vi "FPGA_target_find_stop_output.vi"(5 "start_addr":u32, 7 "number_cmds_in":u32) -> (9 "C0_data":T1, 10 "found":bool, 11 "C1_data":T1, 13 "number_cmds_dup":u32)   [LabVIEW 2014]
doc: "This VI searchs the next stop command following the start address."
uses:
  FPGA_32BitPattern_data_type.ctl
  <vilib>/rvi/Emulation/niFpgaCriticalErrorInLSC.vi
  <vilib>/rvi/Emulation/niFpgaEmulationReportErrorSimple.vi
  <vilib>/rvi/Emulation/niFpgaSctlEmulationGetInTimedLoop.vi
  <vilib>/rvi/Emulation/niFpgaGetClockAttributes.vi
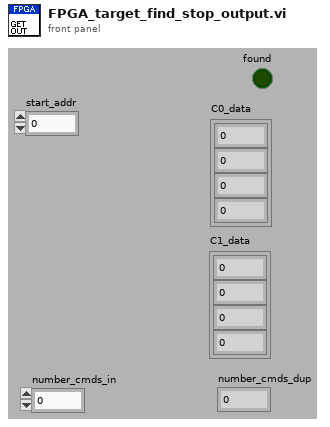
[diagram p1: front panel]
types:
  T1 = typedef "FPGA_32BitPattern_data_type.ctl" = cluster{"port0":u8, "port1":u8, "port2":u8, "port3":u8}
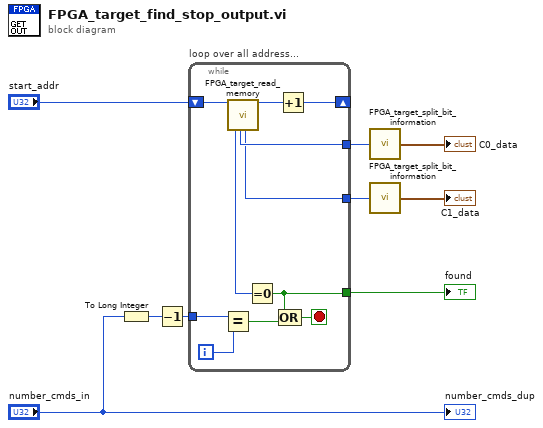
[diagram p0: block diagram]
diagram:
  n1 = To Long Integer(number="number_cmds_in") -> (32bit integer=w7:i32)
  n2 = Decrement(x=w7) -> (x-1=w8:i32)
  n3 = while "loop over all address..." {
    tunnel: w8 -> [w16]
    shift-right: [w14] -> _
    shift-left: "start_addr" -> [w20]
    tunnel: [w12] -> w6
    tunnel: [w11] -> w4
    tunnel: [w10] -> w2
    i -> [w18]
    stop <- w13 stop-if-true
    n4 = Equal?(x=w16, y=w18) -> (x = y?=w15:bool)
    n5 = call "FPGA_target_read_memory.vi"("addr_in"=w20) -> ("data_mem0"=w19:u8, "data_mem1"=w12:u32, "data_mem2"=w11:u32, "addr_dup"=w17:u32)  [unwired: 13 in, 2 out]
    n6 = Equal To 0?(x=w19) -> (x = 0?=w10:bool)
    n7 = Increment(x=w17) -> (x+1=w14:u32)
    n8 = Compound Arithmetic op=OR(w10, w15) -> (w13:bool)
  }
  "found" <- w2
  n9 = call "FPGA_target_split_bit_information.vi"("data in"=w6) -> ("connector_data"=→"C0_data":T1)
  n10 = call "FPGA_target_split_bit_information.vi"("data in"=w4) -> ("connector_data"=→"C1_data":T1)
  "number_cmds_dup" <- "number_cmds_in"
